vi "from string.vi"(8 "error in":errorcluster, 9 "data":string, 10 "version":string, 11 "configuration in":refnum<class "Device Configuration.lvclass">) -> (0 "error out":errorcluster, 3 "configuration out":refnum<class "Device Configuration.lvclass">)   [LabVIEW 2014, in "Device Configuration.lvclass"]
doc: "Provides an interface for loading a module configuration from a file or other serialized data source. It is recommended that all children of this class store data in two sets--data required for its own initialization, and any data required for parent initialization--and that each implementation uses the <b>Call Parent Method</b> primitive to de-serialize parent information."
uses:
  Device Configuration.lvclass
  Device Configuration.lvclass/Device Configuration.ctl
  <vilib>/NI/Configuration Framework/serializable configuration/NISE_CEF_serializable configuration.lvclass
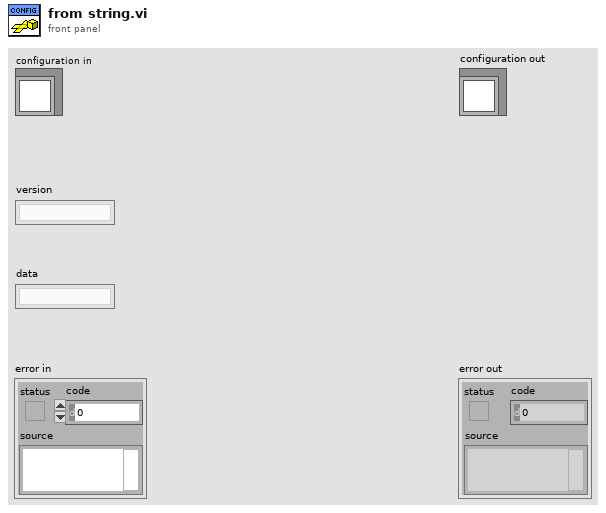
[diagram p1: front panel]
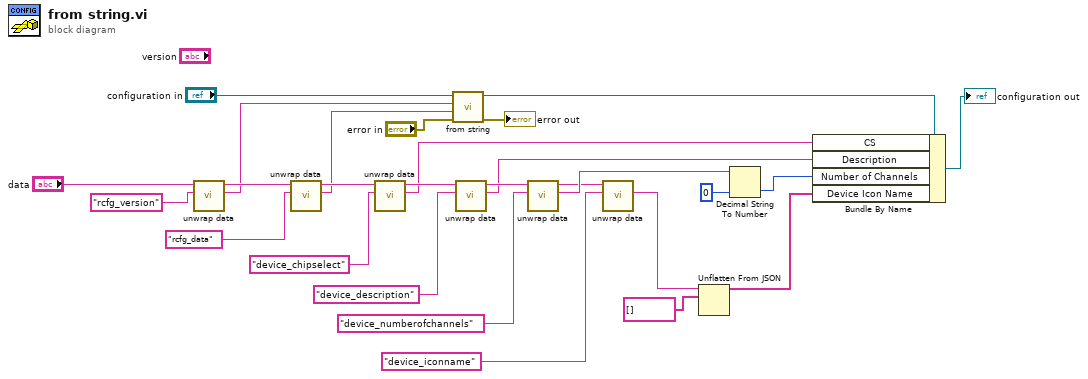
[diagram p0: block diagram]
diagram:
  n1 = call <vilib>:"unwrap data.vi"("identifier"="rcfg_version" ("additional identifier"), "data to unwrap"="data") -> ("unwrapped data"=w17:string, "remaining string"=w26:string)  [unwired: 8 in]
  n2 = call <vilib>:"unwrap data.vi"("identifier"="rcfg_data" ("additional identifier"), "data to unwrap"=w26) -> ("unwrapped data"=w16:string, "remaining string"=w23:string)  [unwired: 8 in]
  n3 = call <vilib>:"unwrap data.vi"("identifier"="device_chipselect" ("additional identifier"), "data to unwrap"=w23) -> ("unwrapped data"=w13:string, "remaining string"=w21:string)  [unwired: 8 in]
  n4 = call-parent "from string.vi"("error in"="error in", "data"=w16, "version"=w17, "configuration in"="configuration in") -> ("error out"=→"error out":errorcluster, "configuration out"=w14:refnum<class "Device Configuration.lvclass">)  [unwired: 6 in]
  n5 = call <vilib>:"unwrap data.vi"("identifier"="device_description", "data to unwrap"=w21) -> ("unwrapped data"=w12:string, "remaining string"=w19:string)  [unwired: 8 in]
  n6 = call <vilib>:"unwrap data.vi"("identifier"="device_numberofchannels" ("data to unwrap"), "data to unwrap"=w19) -> ("unwrapped data"=w11:string, "remaining string"=w6:string)  [unwired: 8 in]
  n7 = call <vilib>:"unwrap data.vi"("identifier"="device_iconname", "data to unwrap"=w6) -> ("unwrapped data"=w3:string)  [unwired: 8 in, 1 out]
  n8 = Unflatten From JSON(JSON string=w3, type and defaults=string[] []) -> (value=w1:string[])  [unwired: 5 in, 1 out]
  n9 = Decimal String To Number(string=w11, default (0L)=u32 0 ("default (0 I32)")) -> (number=w4:u32)  [unwired: 1 in, 1 out]
  n10 = Bundle By Name(cluster=w14, "CS"=w13, "Description"=w12, "Number of Channels"=w4, "Device Icon Name"=w1) -> (→"configuration out":refnum<class "Device Configuration.lvclass">)
